vi "Draw Rays.vi"(6 "Draw Para":T2={"color(black)"=0, "pen"={"Width"=1, "Style"=enum."Solid"}}, 8 "错误输入":errorcluster, 9 "Para":T1, 10 "Center":T3, 11 "Pic in":picture) -> (0 "错误输出":errorcluster, 3 "Pic out":picture)   [LabVIEW 2012, in "Picture Box Tools.lvlib" / "Basic Shape.lvlib"]
uses:
  Basic Shape.lvlib
  Point Custom Control.ctl
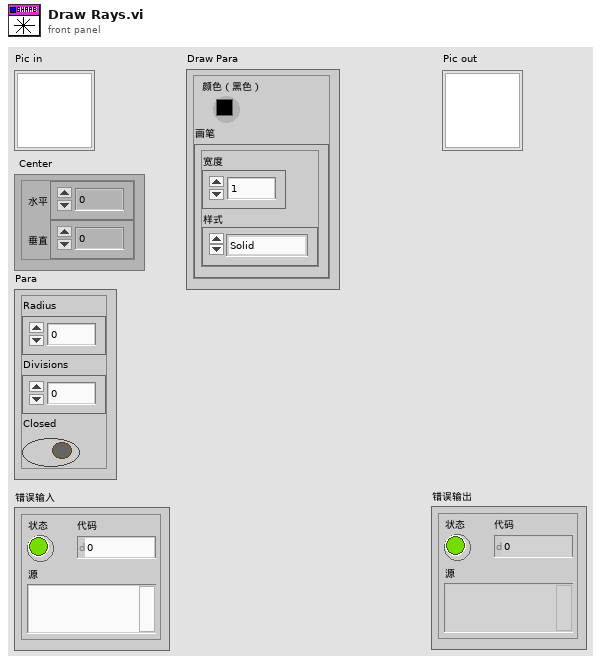
[diagram p1: front panel]
types:
  T1 = cluster{"Radius":i16, "Divisions":i16, "Closed":bool}
  T2 = cluster{"color(black)":u32, "pen":cluster{"Width":u16, "Style":enum32{"Solid", "Dash", "Dot", "DashDot", "DashDotDot"}}}
  T3 = typedef "Picture Box Tools.lvlib/Basic Shape.lvlib/Point Custom Control.ctl" = cluster{"horizontal":i16, "vertical":i16}
  T4 = cluster{"Width":u16, "Style":enum32{"Solid", "Dash", "Dot", "DashDot", "DashDotDot"}}
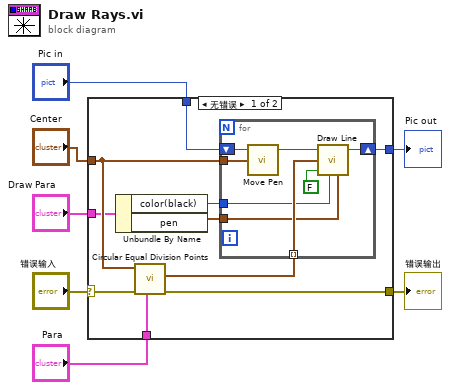
[diagram p0: block diagram]
diagram:
  n1 = case shown="无错误" "错误输入" {
    selector: "错误输入" -> [w17 w27]
    tunnel: [w16 w27] -> w6
    tunnel: "Para" -> [w8 _]
    tunnel: "Center" -> [w12 _]
    tunnel: "Pic in" -> [w14 w26]
    tunnel: [w13 w26] -> w2
    tunnel: "Draw Para" -> [w11 _]
    frame No Error {
      n2 = Unbundle By Name(w11) -> ("color(black)"=w9:u32, "pen"=w10:T4)
      n3 = call "Circular Equal Division Points.vi"("Para"=w8, "错误输入"=w17, "Center"=w12) -> ("错误输出"=w16:errorcluster, "Relative Point Array"=w15:T3[])  [unwired: 6 in, 1 out]
      n4 = for {
        tunnel: w15 -> [w21] mode=indexing
        shift-right: [w22] -> w13
        shift-left: w14 -> [w25]
        tunnel: w12 -> [w23]
        tunnel: w10 -> [w19]
        tunnel: w9 -> [w18]
        n5 = call <vilib>:"Move Pen.vi"("new position"=w23, "picture"=w25) -> ("new picture"=w24:picture)  [unwired: 3 in]
        n6 = call <vilib>:"Draw Line.vi"("picture"=w24, "end point"=w21, "absolute coordinates?(T)"=FALSE, "color(black)"=w18, "pen"=w19) -> ("new picture"=w22:picture)  [unwired: 4 in]
      }
    }
    frame Error {
    }
  }
  "Pic out" <- w2
  "错误输出" <- w6
